vi "Write Allow Mixed.vi"(8 "error in (no error)":errorcluster, 10 "AllowMixed":bool, 11 "MixedCheckbox.lvclass in":refnum<class "MixedCheckbox.lvclass">) -> (0 "error out":errorcluster, 3 "MixedCheckbox.lvclass out":refnum<class "MixedCheckbox.lvclass">)   [LabVIEW 2015, in "MixedCheckbox.lvclass"]
uses:
  MixedCheckbox.lvclass
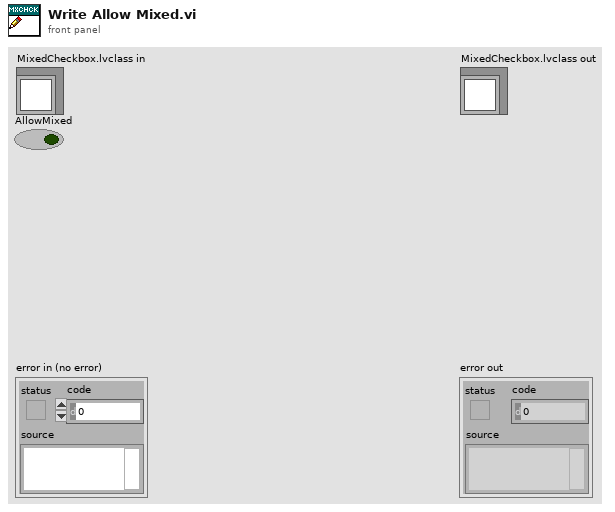
[diagram p1: front panel]
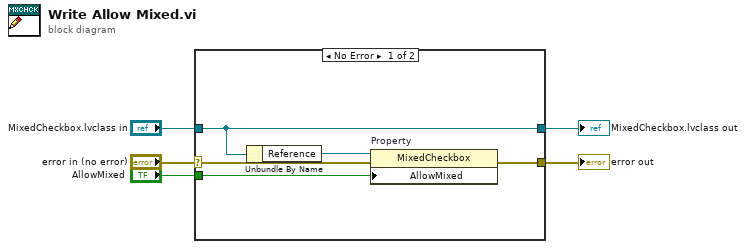
[diagram p0: block diagram]
diagram:
  n1 = case shown="No Error" "error in (no error)" {
    selector: "error in (no error)" -> [w6 w12]
    tunnel: [w10 w12] -> w4
    tunnel: [w8 w11] -> w2
    tunnel: "MixedCheckbox.lvclass in" -> [w8 w11]
    tunnel: "AllowMixed" -> [w9 _]
    frame No Error {
      n2 = Unbundle By Name(w8) -> ("Reference"=w7:refnum<vi>)
      n3 = property on="Property" class="MixedCheckbox"(reference=w7, error in=w6, "AllowMixed"=w9) -> (error out=w10:errorcluster)  [unwired: 1 out]
    }
    frame Error {
    }
  }
  "error out" <- w4
  "MixedCheckbox.lvclass out" <- w2
